vi "Deadzone.vi"(4 "Deadzone":dbl, 6 "Input 4":dbl, 7 "Input 3":dbl, 8 "Input 2":dbl, 9 "Input":dbl) -> (0 "Output 4":dbl, 1 "Output 3":dbl, 2 "Output 2":dbl, 3 "Output":dbl)   [LabVIEW 2013]
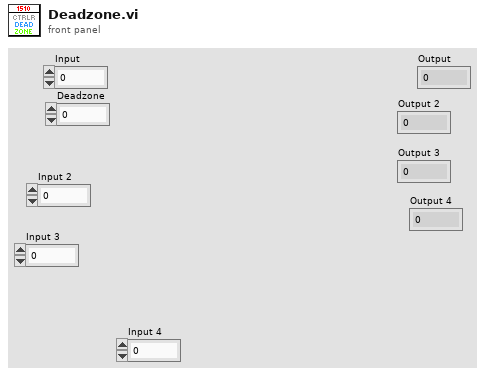
[diagram p1: front panel]
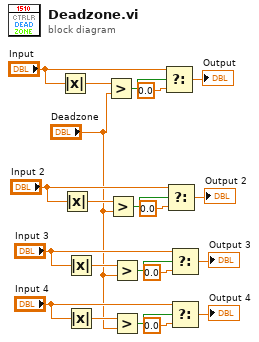
[diagram p0: block diagram]
diagram:
  n1 = Absolute Value(x="Input") -> (abs(x)=w20:dbl)
  n2 = Absolute Value(x="Input 2") -> (abs(x)=w15:dbl)
  n3 = Absolute Value(x="Input 3") -> (abs(x)=w10:dbl)
  n4 = Absolute Value(x="Input 4") -> (abs(x)=w5:dbl)
  n5 = Greater?(x=w20, y="Deadzone") -> (0:w19:bool)
  n6 = Greater?(x=w15, y="Deadzone") -> (0:w14:bool)
  n7 = Greater?(x=w10, y="Deadzone") -> (0:w9:bool)
  n8 = Greater?(x=w5, y="Deadzone") -> (0:w4:bool)
  n9 = Select(t="Input", s=w19, f=0.0) -> (s? t:f=→"Output":dbl)
  n10 = Select(t="Input 2", s=w14, f=0.0) -> (s? t:f=→"Output 2":dbl)
  n11 = Select(t="Input 3", s=w9, f=0.0) -> (s? t:f=→"Output 3":dbl)
  n12 = Select(t="Input 4", s=w4, f=0.0) -> (s? t:f=→"Output 4":dbl)
